vi "Delete LV Object.vi"(7 "error out 2":errorcluster, 10 "reference":refnum<vi>) -> (0 "error out":errorcluster)   [LabVIEW 2018, in "Scripting Tools.lvlib"]
uses:
  Scripting Tools.lvlib
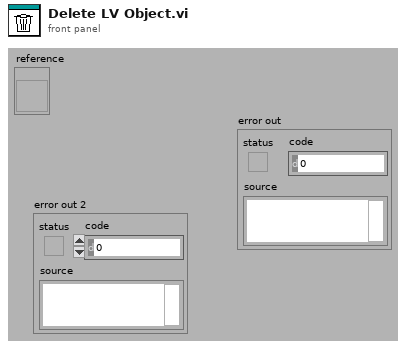
[diagram p1: front panel]
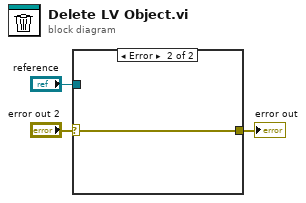
[diagram p0: block diagram]
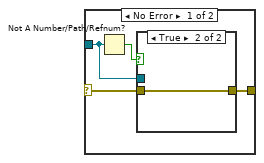
[diagram p2: hidden frame]
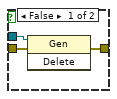
[diagram p3: hidden frame]
diagram:
  n1 = case shown="Error" "error out 2" {
    selector: "error out 2" -> [w5 w12]
    tunnel: [w7 w12] -> w3
    tunnel: "reference" -> [w6 _]
    frame No Error {
      n2 = Not A Number/Path/Refnum?(number/path/refnum=w6) -> (NaN/Path/Refnum?=w4:bool)
      n3 = case shown="True" w4 {
        tunnel: [w10 w11] -> w7
        tunnel: w6 -> [w9 _]
        tunnel: w5 -> [w8 w11]
        frame False {
          n4 = invoke class="Gen" method="Delete"(reference=w9, error in=w8) -> (error out=w10:errorcluster)  [unwired: 1 in, 2 out]
        }
        frame True {
        }
      }
    }
    frame Error {
    }
  }
  "error out" <- w3
